vi "Lab Panel V4.90.vi"() -> ()   [LabVIEW 2013] (continued)
                                n569 = local read "TDMS LAB01-2"() -> (w903:refnum<k34>)
                                n570 = Build Array("Testers Name", "Description", "Set Test Cycles", "T-Rise minutes", "T-Rise Deg C") -> (w893:string[])
                                n571 = Unbundle(w892) -> ("NAME"=w891:string, "DESCRIPTION"=w890:string, "CYCLES"=w889:dbl, "T-RISE mins"=w888:dbl, "T-RISE deg C"=w887:dbl)
                                n572 = Number To Decimal String(number=w889) -> (decimal integer string=w902:string)  [unwired: 1 in]
                                n573 = Number To Decimal String(number=w888) -> (decimal integer string=w901:string)  [unwired: 1 in]
                                n574 = Number To Decimal String(number=w887) -> (decimal integer string=w900:string)  [unwired: 1 in]
                                n575 = Build Array(w891, w890, w902, w901, w900) -> (w899:string[])
                                n576 = TDMS Set Properties(5:w899, 7:w893, 11:w903) -> ()  [unwired: 3 in, 4 out]
                              }
                              frame #3 {
                                n577 = local read "DISP LAB01-2"() -> (w905:T4)
                                n578 = Concatenate Strings("LAB01-2  ", w908) -> (w909:string)
                                n579 = Two Button Dialog(message=w909, 1:w906, 2:w907) -> (T button?=w911:bool)
                                n580 = case shown="True" w911 {
                                tunnel: w905 -> [w918 w919]
                                tunnel: [w918 w919] -> w915
                                tunnel: [w917 w920] -> w914
                                tunnel: [w916 w920] -> w913
                                frame False {
                                n581 = Unbundle(w918) -> ("CYCLE"=w917:dbl, "MINS"=w916:dbl)  [unwired: 1 out]
                                }
                                frame True {
                                w920 = 0.0
                                }
                                }
                                n582 = Bundle(cluster=w915, "CYCLE"=w914, "MINS"=w913, "STATUS"="RUN") -> (w904:T4)
                                n583 = local write "DISP LAB01-2"(w904) -> ()
                              }
                              frame #4 {
                                n584 = local read "TEMP START LAB01-2"() -> (w923:cluster{"TL":dbl, "TN":dbl})
                                n585 = Bundle(cluster=w923, "TL"=w921, "TN"=w921) -> (w922:cluster{"TL":dbl, "TN":dbl})
                                n586 = local write "TEMP START LAB01-2"(w922) -> ()
                              }
                            }
                          }
                        }
                      }
                    }
                  }
                }
              }
              event "RUN LAB02-1": Value Change {
                n587 = event-data() -> ("NewVal"=w929:bool)  [unwired: 1 in, 5 out]
                n588 = local read "SIG LAB02-1"() -> (w925:T2)
                n589 = case shown="True" w929 {
                  tunnel: w935 -> [_ w973]
                  tunnel: w934 -> [_ w972]
                  tunnel: w932 -> [w937 w971]
                  tunnel: w933 -> [_ w970]
                  tunnel: w931 -> [_ w969]
                  tunnel: [w936 w968] -> w930
                  tunnel: w928 -> [_ w967]
                  tunnel: w927 -> [_ w966]
                  tunnel: w926 -> [_ w965]
                  tunnel: w925 -> [_ w964]
                  tunnel: w924 -> [_ w963]
                  frame False {
                    # "stop test"
                    n590 = stacked-sequence {
                      tunnel: w937 -> [w946 _]
                      tunnel: [w938 _] -> w936
                      frame #0 {
                        n591 = local read "DISP LAB02-1"() -> (w945:T4)
                        n592 = Unbundle(w945) -> ("CYCLE"=w943:dbl, "MINS"=w944:dbl)  [unwired: 1 out]
                        n593 = case shown="\"CYCLE TEST\"" w946 {
                          tunnel: w944 -> [_ _ w953]
                          tunnel: w943 -> [w951 w952 _]
                          tunnel: [w951 w952 w953] -> w942
                          frame "CHART TEST", Default {
                          }
                          frame "CYCLE TEST" {
                          }
                          frame "T-RISE TEST" {
                          }
                        }
                        n594 = local read "TDMS LAB02-1"() -> (w950:refnum<k34>)
                        n595 = Build Array("STOPPED") -> (w947:string[])
                        n596 = Build Array(w942) -> (w941:dbl[])
                        n597 = TDMS Write(0:w950, 5:"TEST RESULT", 7:w947, 9:w941) -> (4:w939:refnum<k34>, 15:w940:errorcluster)  [unwired: 2 in, 2 out]
                        n598 = TDMS Close(8:w940, 11:w939) -> (0:w938:errorcluster)  [unwired: 1 out]
                      }
                      frame #1 {
                        n599 = local read "DISP LAB02-1"() -> (w957:T4)
                        n600 = stacked-sequence {
                          tunnel: "LAB02-1" -> [w959 w961]
                          frame #0 {
                            n601 = call "sub vi - defrag tdms v1.vi"("panel id"=w959) -> ("error out"=w958:errorcluster)  [unwired: 10 in]
                            n602 = local write "data file error"(w958) -> ()
                          }
                          frame #1 {
                            n603 = local write "RESULT LAB02-1"(FALSE) -> ()
                            n604 = call "Save data file (stop) v3.vi"("panel id"=w961) -> ("network file save error"=w960:errorcluster)  [unwired: 9 in, 1 out]
                            n605 = local write "data file error"(w960) -> ()
                          }
                        }
                        n606 = Bundle(cluster=w957, "STATUS"="STOP") -> (w955:T4)  [unwired: 2 in]
                        n607 = local write "DISP LAB02-1"(w955) -> ()
                      }
                    }
                  }
                  frame True {
                    n608 = stacked-sequence {
                      seq-local: [w975 _] -> [_ w979]
                      tunnel: w973 -> [_ w989]
                      tunnel: w972 -> [_ w988]
                      tunnel: w971 -> [_ w987]
                      tunnel: w970 -> [_ w986]
                      tunnel: w969 -> [_ w985]
                      tunnel: [_ w984] -> w968
                      tunnel: w967 -> [_ w983]
                      tunnel: w966 -> [_ w982]
                      tunnel: w965 -> [_ w981]
                      tunnel: w964 -> [w974 w980]
                      tunnel: w963 -> [_ w978]
                      frame #0 {
                        n609 = Unbundle(w974) -> ("AMPS"=w977:dbl)  [unwired: 4 out]
                        n610 = call "Check For Amps on v1.vi"("ID"="LAB02-1", "amps"=w977) -> ("amps"=w975:bool)  [unwired: 9 in]
                      }
                      frame #1 {
                        n611 = case shown="True" w979 {
                          tunnel: w989 -> [_ w1002]
                          tunnel: w988 -> [_ w1001]
                          tunnel: w987 -> [_ w1000]
                          tunnel: w986 -> [_ w999]
                          tunnel: w985 -> [_ w998]
                          tunnel: [errorcluster {"status"=FALSE, "code"=0, "source"=""} ("error out") w997] -> w984
                          tunnel: w983 -> [_ w996]
                          tunnel: w982 -> [_ w995]
                          tunnel: w981 -> [_ w994]
                          tunnel: w980 -> [_ w993]
                          tunnel: w978 -> [_ w992]
                          frame False {
                            w991 = FALSE
                            n612 = local write "RUN LAB02-1"(w991) -> ()
                            n613 = local write "run lab02-1"(w991) -> ()
                          }
                          frame True {
                            n614 = stacked-sequence {
                              seq-local: [w1003 _ _ _ _] -> [_ w1027 _ _ _]
                              tunnel: w1002 -> [w1008 _ _ _ _]
                              tunnel: w1001 -> [w1005 _ _ _ _]
                              tunnel: w1000 -> [w1018 _ _ _ _]
                              tunnel: w999 -> [w1011 _ _ _ _]
                              tunnel: w998 -> [w1006 _ _ _ _]
                              tunnel: [_ w1022 _ _ _] -> w997
                              tunnel: w996 -> [_ _ _ w1048 _]
                              tunnel: w995 -> [_ _ _ w1047 _]
                              tunnel: w994 -> [_ _ _ w1046 _]
                              tunnel: w993 -> [_ _ _ _ _]
                              tunnel: w992 -> [_ _ _ _ w1062]
                              frame #0 {
                                w1004 = "\\"
                                n615 = local read "SET LAB02-1"() -> (w1013:T5)
                                n616 = case shown="\"CYCLE TEST\"" w1018 {
                                tunnel: ["L02-1-CHART TEST-" "L02-1-CYCLE TEST-" "L02-1-T-RISE TEST-"] -> w1014
                                frame "CHART TEST", Default {
                                }
                                frame "CYCLE TEST" {
                                }
                                frame "T-RISE TEST" {
                                }
                                }
                                n617 = Unbundle(w1013) -> ("DESCRIPTION"=w1012:string)  [unwired: 4 out]
                                n618 = Concatenate Strings(w1008, "\\", w1006, w1004, w1005, w1004) -> (w1015:string)
                                n619 = String To Path(string=w1015) -> (path=w1017:path)
                                n620 = Concatenate Strings(w1015, w1014, w1012, "-", w1011, ".tdms") -> (w1003:string)
                                n621 = Create Folder(path (use dialog)=w1017) -> (error out=w1016:errorcluster)  [unwired: 2 in, 2 out]
                                n622 = global write "Global 1.vi" "LAB02-1 FILE"(w1003) -> ()
                                n623 = call <vilib>:"Clear Errors.vi"("error in (no error)"=w1016) -> ()  [unwired: 6 in, 1 out]
                              }
                              frame #1 {
                                (unwired) FALSE
                                n624 = String To Path(string=w1027) -> (path=w1023:path)
                                n625 = TDMS Open(6:FALSE, 10:T20."create or replace" ("operation (0:open)"), 11:w1023) -> (0:w1022:errorcluster, 3:→"TDMS LAB02-1":refnum<k34>)  [unwired: 4 in]
                              }
                              frame #2 {
                                n626 = local read "SET LAB02-1"() -> (w1033:T5)
                                n627 = local read "TDMS LAB02-1"() -> (w1044:refnum<k34>)
                                n628 = Build Array("Testers Name", "Description", "Set Test Cycles", "T-Rise minutes", "T-Rise Deg C") -> (w1034:string[])
                                n629 = Unbundle(w1033) -> ("NAME"=w1032:string, "DESCRIPTION"=w1031:string, "CYCLES"=w1030:dbl, "T-RISE mins"=w1029:dbl, "T-RISE deg C"=w1028:dbl)
                                n630 = Number To Decimal String(number=w1030) -> (decimal integer string=w1043:string)  [unwired: 1 in]
                                n631 = Number To Decimal String(number=w1029) -> (decimal integer string=w1042:string)  [unwired: 1 in]
                                n632 = Number To Decimal String(number=w1028) -> (decimal integer string=w1041:string)  [unwired: 1 in]
                                n633 = Build Array(w1032, w1031, w1043, w1042, w1041) -> (w1040:string[])
                                n634 = TDMS Set Properties(5:w1040, 7:w1034, 11:w1044) -> ()  [unwired: 3 in, 4 out]
                              }
                              frame #3 {
                                n635 = local read "DISP LAB02-1"() -> (w1049:T4)
                                n636 = Concatenate Strings("LAB02-1  ", w1048) -> (w1050:string)
                                n637 = Two Button Dialog(message=w1050, 1:w1046, 2:w1047) -> (T button?=w1052:bool)
                                n638 = case shown="True" w1052 {
                                tunnel: w1049 -> [w1059 w1060]
                                tunnel: [w1059 w1060] -> w1056
                                tunnel: [w1058 w1061] -> w1055
                                tunnel: [w1057 w1061] -> w1054
                                frame False {
                                n639 = Unbundle(w1059) -> ("CYCLE"=w1058:dbl, "MINS"=w1057:dbl)  [unwired: 1 out]
                                }
                                frame True {
                                w1061 = 0.0
                                }
                                }
                                n640 = Bundle(cluster=w1056, "CYCLE"=w1055, "MINS"=w1054, "STATUS"="RUN") -> (w1045:T4)
                                n641 = local write "DISP LAB02-1"(w1045) -> ()
                              }
                              frame #4 {
                                n642 = local read "TEMP START LAB02-1"() -> (w1064:cluster{"TL":dbl, "TN":dbl})
                                n643 = Bundle(cluster=w1064, "TL"=w1062, "TN"=w1062) -> (w1063:cluster{"TL":dbl, "TN":dbl})
                                n644 = local write "TEMP START LAB02-1"(w1063) -> ()
                              }
                            }
                          }
                        }
                      }
                    }
                  }
                }
                n645 = local write "run lab02-1"(w929) -> ()
              }
              event "RUN LAB02-2": Value Change {
                n646 = event-data() -> ("NewVal"=w1069:bool)  [unwired: 1 in, 5 out]
                n647 = local write "run lab02-2"(w1069) -> ()
                n648 = case shown="True" w1069 {
                  tunnel: w1075 -> [_ w1113]
                  tunnel: w1074 -> [_ w1112]
                  tunnel: w1072 -> [w1077 w1111]
                  tunnel: w1073 -> [_ w1110]
                  tunnel: w1071 -> [_ w1109]
                  tunnel: [w1076 w1108] -> w1070
                  tunnel: w1068 -> [_ w1107]
                  tunnel: w1067 -> [_ w1106]
                  tunnel: w1066 -> [_ w1105]
                  tunnel: w1065 -> [_ w1103]
                  frame False {
                    # "stop test"
                    n649 = stacked-sequence {
                      tunnel: w1077 -> [w1086 _]
                      tunnel: [w1078 _] -> w1076
                      frame #0 {
                        n650 = local read "DISP LAB02-2"() -> (w1085:T4)
                        n651 = Unbundle(w1085) -> ("CYCLE"=w1083:dbl, "MINS"=w1084:dbl)  [unwired: 1 out]
                        n652 = case shown="\"CYCLE TEST\"" w1086 {
                          tunnel: w1084 -> [_ _ w1093]
                          tunnel: w1083 -> [w1091 w1092 _]
                          tunnel: [w1091 w1092 w1093] -> w1082
                          frame "CHART TEST", Default {
                          }
                          frame "CYCLE TEST" {
                          }
                          frame "T-RISE TEST" {
                          }
                        }
                        n653 = local read "TDMS LAB02-2"() -> (w1090:refnum<k34>)
                        n654 = Build Array("STOPPED") -> (w1087:string[])
                        n655 = Build Array(w1082) -> (w1081:dbl[])
                        n656 = TDMS Write(0:w1090, 5:"TEST RESULT", 7:w1087, 9:w1081) -> (4:w1079:refnum<k34>, 15:w1080:errorcluster)  [unwired: 2 in, 2 out]
                        n657 = TDMS Close(8:w1080, 11:w1079) -> (0:w1078:errorcluster)  [unwired: 1 out]
                      }
                      frame #1 {
                        n658 = local read "DISP LAB02-2"() -> (w1097:T4)
                        n659 = stacked-sequence {
                          tunnel: "LAB02-2" -> [w1099 w1101]
                          frame #0 {
                            n660 = call "sub vi - defrag tdms v1.vi"("panel id"=w1099) -> ("error out"=w1098:errorcluster)  [unwired: 10 in]
                            n661 = local write "data file error"(w1098) -> ()
                          }
                          frame #1 {
                            n662 = call "Save data file (stop) v3.vi"("panel id"=w1101) -> ("network file save error"=w1100:errorcluster)  [unwired: 9 in, 1 out]
                            n663 = local write "RESULT LAB02-2"(FALSE) -> ()
                            n664 = local write "data file error"(w1100) -> ()
                          }
                        }
                        n665 = Bundle(cluster=w1097, "STATUS"="STOP") -> (w1095:T4)  [unwired: 2 in]
                        n666 = local write "DISP LAB02-2"(w1095) -> ()
                      }
                    }
                  }
                  frame True {
                    n667 = local read "SIG LAB02-2"() -> (w1104:T2)
                    n668 = stacked-sequence {
                      seq-local: [w1115 _] -> [_ w1119]
                      tunnel: w1113 -> [_ w1129]
                      tunnel: w1112 -> [_ w1128]
                      tunnel: w1111 -> [_ w1127]
                      tunnel: w1110 -> [_ w1126]
                      tunnel: w1109 -> [_ w1125]
                      tunnel: [_ w1124] -> w1108
                      tunnel: w1107 -> [_ w1123]
                      tunnel: w1106 -> [_ w1122]
                      tunnel: w1105 -> [_ w1121]
                      tunnel: w1104 -> [w1114 w1120]
                      tunnel: w1103 -> [_ w1118]
                      frame #0 {
                        n669 = Unbundle(w1114) -> ("AMPS"=w1117:dbl)  [unwired: 4 out]
                        n670 = call "Check For Amps on v1.vi"("ID"="LAB02-2", "amps"=w1117) -> ("amps"=w1115:bool)  [unwired: 9 in]
                      }
                      frame #1 {
                        n671 = case shown="True" w1119 {
                          tunnel: w1129 -> [_ w1142]
                          tunnel: w1128 -> [_ w1141]
                          tunnel: w1127 -> [_ w1140]
                          tunnel: w1126 -> [_ w1139]
                          tunnel: w1125 -> [_ w1138]
                          tunnel: [errorcluster {"status"=FALSE, "code"=0, "source"=""} ("error out") w1137] -> w1124
                          tunnel: w1123 -> [_ w1136]
                          tunnel: w1122 -> [_ w1135]
                          tunnel: w1121 -> [_ w1134]
                          tunnel: w1120 -> [_ w1133]
                          tunnel: w1118 -> [_ w1132]
                          frame False {
                            w1130 = FALSE
                            n672 = local write "RUN LAB02-2"(w1130) -> ()
                            n673 = local write "run lab02-2"(w1130) -> ()
                          }
                          frame True {
                            n674 = stacked-sequence {
                              seq-local: [w1143 _ _ _ _] -> [_ w1167 _ _ _]
                              tunnel: w1142 -> [w1148 _ _ _ _]
                              tunnel: w1141 -> [w1145 _ _ _ _]
                              tunnel: w1140 -> [w1158 _ _ _ _]
                              tunnel: w1139 -> [w1151 _ _ _ _]
                              tunnel: w1138 -> [w1146 _ _ _ _]
                              tunnel: [_ w1162 _ _ _] -> w1137
                              tunnel: w1136 -> [_ _ _ w1188 _]
                              tunnel: w1135 -> [_ _ _ w1187 _]
                              tunnel: w1134 -> [_ _ _ w1186 _]
                              tunnel: w1133 -> [_ _ _ _ _]
                              tunnel: w1132 -> [_ _ _ _ w1202]
                              frame #0 {
                                w1144 = "\\"
                                n675 = local read "SET LAB02-2"() -> (w1153:T5)
                                n676 = case shown="\"CYCLE TEST\"" w1158 {
                                tunnel: ["L02-2-CHART TEST-" "L02-2-CYCLE TEST-" "L02-2-T-RISE TEST-"] -> w1154
                                frame "CHART TEST", Default {
                                }
                                frame "CYCLE TEST" {
                                }
                                frame "T-RISE TEST" {
                                }
                                }
                                n677 = Unbundle(w1153) -> ("DESCRIPTION"=w1152:string)  [unwired: 4 out]
                                n678 = Concatenate Strings(w1148, "\\", w1146, w1144, w1145, w1144) -> (w1155:string)
                                n679 = String To Path(string=w1155) -> (path=w1157:path)
                                n680 = Concatenate Strings(w1155, w1154, w1152, "-", w1151, ".tdms") -> (w1143:string)
                                n681 = Create Folder(path (use dialog)=w1157) -> (error out=w1156:errorcluster)  [unwired: 2 in, 2 out]
                                n682 = global write "Global 1.vi" "LAB02-2 FILE"(w1143) -> ()
                                n683 = call <vilib>:"Clear Errors.vi"("error in (no error)"=w1156) -> ()  [unwired: 6 in, 1 out]
                              }
                              frame #1 {
                                (unwired) FALSE
                                n684 = String To Path(string=w1167) -> (path=w1163:path)
                                n685 = TDMS Open(6:FALSE, 10:T20."create or replace" ("operation (0:open)"), 11:w1163) -> (0:w1162:errorcluster, 3:→"TDMS LAB02-2":refnum<k34>)  [unwired: 4 in]
                              }
                              frame #2 {
                                n686 = local read "SET LAB02-2"() -> (w1173:T5)
                                n687 = local read "TDMS LAB02-2"() -> (w1184:refnum<k34>)
                                n688 = Build Array("Testers Name", "Description", "Set Test Cycles", "T-Rise minutes", "T-Rise Deg C") -> (w1174:string[])
                                n689 = Unbundle(w1173) -> ("NAME"=w1172:string, "DESCRIPTION"=w1171:string, "CYCLES"=w1170:dbl, "T-RISE mins"=w1169:dbl, "T-RISE deg C"=w1168:dbl)
                                n690 = Number To Decimal String(number=w1170) -> (decimal integer string=w1183:string)  [unwired: 1 in]
                                n691 = Number To Decimal String(number=w1169) -> (decimal integer string=w1182:string)  [unwired: 1 in]
                                n692 = Number To Decimal String(number=w1168) -> (decimal integer string=w1181:string)  [unwired: 1 in]
                                n693 = Build Array(w1172, w1171, w1183, w1182, w1181) -> (w1180:string[])
                                n694 = TDMS Set Properties(5:w1180, 7:w1174, 11:w1184) -> ()  [unwired: 3 in, 4 out]
                              }
                              frame #3 {
                                n695 = local read "DISP LAB02-2"() -> (w1189:T4)
                                n696 = Concatenate Strings("LAB02-2  ", w1188) -> (w1190:string)
                                n697 = Two Button Dialog(message=w1190, 1:w1186, 2:w1187) -> (T button?=w1192:bool)
                                n698 = case shown="True" w1192 {
                                tunnel: w1189 -> [w1199 w1200]
                                tunnel: [w1199 w1200] -> w1196
                                tunnel: [w1198 w1201] -> w1195
                                tunnel: [w1197 w1201] -> w1194
                                frame False {
                                n699 = Unbundle(w1199) -> ("CYCLE"=w1198:dbl, "MINS"=w1197:dbl)  [unwired: 1 out]
                                }
                                frame True {
                                w1201 = 0.0
                                }
                                }
                                n700 = Bundle(cluster=w1196, "CYCLE"=w1195, "MINS"=w1194, "STATUS"="RUN") -> (w1185:T4)
                                n701 = local write "DISP LAB02-2"(w1185) -> ()
                              }
                              frame #4 {
                                n702 = local read "TEMP START LAB02-2"() -> (w1204:cluster{"TL":dbl, "TN":dbl})
                                n703 = Bundle(cluster=w1204, "TL"=w1202, "TN"=w1202) -> (w1203:cluster{"TL":dbl, "TN":dbl})
                                n704 = local write "TEMP START LAB02-2"(w1203) -> ()
                              }
                            }
                          }
                        }
                      }
                    }
                  }
                }
              }
              event "RUN LAB03-1": Value Change {
                n705 = event-data() -> ("NewVal"=w1209:bool)  [unwired: 1 in, 5 out]
                n706 = local write "run lab03-1"(w1209) -> ()
                n707 = case shown="True" w1209 {
                  tunnel: w1215 -> [_ w1253]
                  tunnel: w1214 -> [_ w1252]
                  tunnel: w1212 -> [w1217 w1251]
                  tunnel: w1213 -> [_ w1250]
                  tunnel: w1211 -> [_ w1249]
                  tunnel: [w1216 w1248] -> w1210
                  tunnel: w1208 -> [_ w1247]
                  tunnel: w1207 -> [_ w1246]
                  tunnel: w1206 -> [_ w1245]
                  tunnel: w1205 -> [_ w1243]
                  frame False {
                    # "stop test"
                    n708 = stacked-sequence {
                      tunnel: w1217 -> [w1226 _]
                      tunnel: [w1218 _] -> w1216
                      frame #0 {
                        n709 = local read "DISP LAB03-1"() -> (w1225:T4)
                        n710 = Unbundle(w1225) -> ("CYCLE"=w1223:dbl, "MINS"=w1224:dbl)  [unwired: 1 out]
                        n711 = case shown="\"CYCLE TEST\"" w1226 {
                          tunnel: w1224 -> [_ _ w1233]
                          tunnel: w1223 -> [w1231 w1232 _]
                          tunnel: [w1231 w1232 w1233] -> w1222
                          frame "CHART TEST", Default {
                          }
                          frame "CYCLE TEST" {
                          }
                          frame "T-RISE TEST" {
                          }
                        }
                        n712 = local read "TDMS LAB03-1"() -> (w1230:refnum<k34>)
                        n713 = Build Array("STOPPED") -> (w1227:string[])
                        n714 = Build Array(w1222) -> (w1221:dbl[])
                        n715 = TDMS Write(0:w1230, 5:"TEST RESULT", 7:w1227, 9:w1221) -> (4:w1219:refnum<k34>, 15:w1220:errorcluster)  [unwired: 2 in, 2 out]
                        n716 = TDMS Close(8:w1220, 11:w1219) -> (0:w1218:errorcluster)  [unwired: 1 out]
                      }
                      frame #1 {
                        n717 = local read "DISP LAB03-1"() -> (w1237:T4)
                        n718 = stacked-sequence {
                          tunnel: "LAB03-1" -> [w1239 w1241]
                          frame #0 {
                            n719 = call "sub vi - defrag tdms v1.vi"("panel id"=w1239) -> ("error out"=w1238:errorcluster)  [unwired: 10 in]
                            n720 = local write "data file error"(w1238) -> ()
                          }
                          frame #1 {
                            n721 = call "Save data file (stop) v3.vi"("panel id"=w1241) -> ("network file save error"=w1240:errorcluster)  [unwired: 9 in, 1 out]
                            n722 = local write "RESULT LAB03-1"(FALSE) -> ()
                            n723 = local write "data file error"(w1240) -> ()
                          }
                        }
                        n724 = Bundle(cluster=w1237, "STATUS"="STOP") -> (w1235:T4)  [unwired: 2 in]
                        n725 = local write "DISP LAB03-1"(w1235) -> ()
                      }
                    }
                  }
                  frame True {
                    n726 = local read "SIG LAB03-1"() -> (w1244:T2)
                    n727 = stacked-sequence {
                      seq-local: [w1255 _] -> [_ w1259]
                      tunnel: w1253 -> [_ w1269]
                      tunnel: w1252 -> [_ w1268]
                      tunnel: w1251 -> [_ w1267]
                      tunnel: w1250 -> [_ w1266]
                      tunnel: w1249 -> [_ w1265]
                      tunnel: [_ w1264] -> w1248
                      tunnel: w1247 -> [_ w1263]
                      tunnel: w1246 -> [_ w1262]
                      tunnel: w1245 -> [_ w1261]
                      tunnel: w1244 -> [w1254 w1260]
                      tunnel: w1243 -> [_ w1258]
                      frame #0 {
                        n728 = Unbundle(w1254) -> ("AMPS"=w1257:dbl)  [unwired: 4 out]
                        n729 = call "Check For Amps on v1.vi"("ID"="LAB03-1", "amps"=w1257) -> ("amps"=w1255:bool)  [unwired: 9 in]
                      }
                      frame #1 {
                        n730 = case shown="True" w1259 {
                          tunnel: w1269 -> [_ w1282]
                          tunnel: w1268 -> [_ w1281]
                          tunnel: w1267 -> [_ w1280]
                          tunnel: w1266 -> [_ w1279]
                          tunnel: w1265 -> [_ w1278]
                          tunnel: [errorcluster {"status"=FALSE, "code"=0, "source"=""} ("error out") w1277] -> w1264
                          tunnel: w1263 -> [_ w1276]
                          tunnel: w1262 -> [_ w1275]
                          tunnel: w1261 -> [_ w1274]
                          tunnel: w1260 -> [_ w1273]
                          tunnel: w1258 -> [_ w1272]
                          frame False {
                            w1270 = FALSE
                            n731 = local write "RUN LAB03-1"(w1270) -> ()
                            n732 = local write "run lab03-1"(w1270) -> ()
                          }
                          frame True {
                            n733 = stacked-sequence {
                              seq-local: [w1283 _ _ _ _] -> [_ w1307 _ _ _]
                              tunnel: w1282 -> [w1288 _ _ _ _]
                              tunnel: w1281 -> [w1285 _ _ _ _]
                              tunnel: w1280 -> [w1298 _ _ _ _]
                              tunnel: w1279 -> [w1291 _ _ _ _]
                              tunnel: w1278 -> [w1286 _ _ _ _]
                              tunnel: [_ w1302 _ _ _] -> w1277
                              tunnel: w1276 -> [_ _ _ w1327 _]
                              tunnel: w1275 -> [_ _ _ w1326 _]
                              tunnel: w1274 -> [_ _ _ w1325 _]
                              tunnel: w1273 -> [_ _ _ _ _]
                              tunnel: w1272 -> [_ _ _ _ w1342]
                              frame #0 {
                                w1284 = "\\"
                                n734 = local read "SET LAB03-1"() -> (w1293:T5)
                                n735 = case shown="\"T-RISE TEST\"" w1298 {
                                tunnel: ["L03-1-CHART TEST-" "L03-1-CYCLE TEST-" "L03-1-T-RISE TEST-"] -> w1294
                                frame "CHART TEST", Default {
                                }
                                frame "CYCLE TEST" {
                                }
                                frame "T-RISE TEST" {
                                }
                                }
                                n736 = Unbundle(w1293) -> ("DESCRIPTION"=w1292:string)  [unwired: 4 out]
                                n737 = Concatenate Strings(w1288, "\\", w1286, w1284, w1285, w1284) -> (w1295:string)
                                n738 = String To Path(string=w1295) -> (path=w1297:path)
                                n739 = Concatenate Strings(w1295, w1294, w1292, "-", w1291, ".tdms") -> (w1283:string)
                                n740 = Create Folder(path (use dialog)=w1297) -> (error out=w1296:errorcluster)  [unwired: 2 in, 2 out]
                                n741 = global write "Global 1.vi" "LAB03-1 FILE"(w1283) -> ()
                                n742 = call <vilib>:"Clear Errors.vi"("error in (no error)"=w1296) -> ()  [unwired: 6 in, 1 out]
                              }
                              frame #1 {
                                (unwired) FALSE
                                n743 = String To Path(string=w1307) -> (path=w1303:path)
                                n744 = TDMS Open(6:FALSE, 10:T20."create or replace" ("operation (0:open)"), 11:w1303) -> (0:w1302:errorcluster, 3:→"TDMS LAB03-1":refnum<k34>)  [unwired: 4 in]
                              }
                              frame #2 {
                                n745 = local read "SET LAB03-1"() -> (w1313:T5)
                                n746 = local read "TDMS LAB03-1"() -> (w1324:refnum<k34>)
                                n747 = Build Array("Testers Name", "Description", "Set Test Cycles", "T-Rise minutes", "T-Rise Deg C") -> (w1314:string[])
                                n748 = Unbundle(w1313) -> ("NAME"=w1312:string, "DESCRIPTION"=w1311:string, "CYCLES"=w1310:dbl, "T-RISE mins"=w1309:dbl, "T-RISE deg C"=w1308:dbl)
                                n749 = Number To Decimal String(number=w1310) -> (decimal integer string=w1323:string)  [unwired: 1 in]
                                n750 = Number To Decimal String(number=w1309) -> (decimal integer string=w1322:string)  [unwired: 1 in]
                                n751 = Number To Decimal String(number=w1308) -> (decimal integer string=w1321:string)  [unwired: 1 in]
                                n752 = Build Array(w1312, w1311, w1323, w1322, w1321) -> (w1320:string[])
                                n753 = TDMS Set Properties(5:w1320, 7:w1314, 11:w1324) -> ()  [unwired: 3 in, 4 out]
                              }
                              frame #3 {
                                n754 = local read "DISP LAB03-1"() -> (w1329:T4)
                                n755 = Concatenate Strings("LAB03-1  ", w1327) -> (w1330:string)
                                n756 = Two Button Dialog(message=w1330, 1:w1325, 2:w1326) -> (T button?=w1332:bool)
                                n757 = case shown="True" w1332 {
                                tunnel: w1329 -> [w1339 w1340]
                                tunnel: [w1339 w1340] -> w1336
                                tunnel: [w1338 w1341] -> w1335
                                tunnel: [w1337 w1341] -> w1334
                                frame False {
                                n758 = Unbundle(w1339) -> ("CYCLE"=w1338:dbl, "MINS"=w1337:dbl)  [unwired: 1 out]
                                }
                                frame True {
                                w1341 = 0.0
                                }
                                }
                                n759 = Bundle(cluster=w1336, "CYCLE"=w1335, "MINS"=w1334, "STATUS"="RUN") -> (w1328:T4)
                                n760 = local write "DISP LAB03-1"(w1328) -> ()
                              }
                              frame #4 {
                                n761 = local read "TEMP START LAB03-1"() -> (w1344:cluster{"TL":dbl, "TN":dbl})
                                n762 = Bundle(cluster=w1344, "TL"=w1342, "TN"=w1342) -> (w1343:cluster{"TL":dbl, "TN":dbl})
                                n763 = local write "TEMP START LAB03-1"(w1343) -> ()
                              }
                            }
                          }
                        }
                      }
                    }
                  }
                }
              }
              event "RUN LAB03-2": Value Change {
                n764 = event-data() -> ("NewVal"=w1349:bool)  [unwired: 1 in, 5 out]
                n765 = local write "run lab03-2"(w1349) -> ()
                n766 = case shown="True" w1349 {
                  tunnel: w1355 -> [_ w1393]
                  tunnel: w1354 -> [_ w1392]
                  tunnel: w1352 -> [w1357 w1391]
                  tunnel: w1353 -> [_ w1390]
                  tunnel: w1351 -> [_ w1389]
                  tunnel: [w1356 w1388] -> w1350
                  tunnel: w1348 -> [_ w1387]
                  tunnel: w1347 -> [_ w1386]
                  tunnel: w1346 -> [_ w1385]
                  tunnel: w1345 -> [_ w1383]
                  frame False {
                    # "stop test"
                    n767 = stacked-sequence {
                      tunnel: w1357 -> [w1366 _]
                      tunnel: [w1358 _] -> w1356
                      frame #0 {
                        n768 = local read "DISP LAB03-2"() -> (w1365:T4)
                        n769 = Unbundle(w1365) -> ("CYCLE"=w1363:dbl, "MINS"=w1364:dbl)  [unwired: 1 out]
                        n770 = case shown="\"CYCLE TEST\"" w1366 {
                          tunnel: w1364 -> [_ _ w1373]
                          tunnel: w1363 -> [w1371 w1372 _]
                          tunnel: [w1371 w1372 w1373] -> w1362
                          frame "CHART TEST", Default {
                          }
                          frame "CYCLE TEST" {
                          }
                          frame "T-RISE TEST" {
                          }
                        }
                        n771 = local read "TDMS LAB03-2"() -> (w1370:refnum<k34>)
                        n772 = Build Array("STOPPED") -> (w1367:string[])
                        n773 = Build Array(w1362) -> (w1361:dbl[])
                        n774 = TDMS Write(0:w1370, 5:"TEST RESULT", 7:w1367, 9:w1361) -> (4:w1359:refnum<k34>, 15:w1360:errorcluster)  [unwired: 2 in, 2 out]
                        n775 = TDMS Close(8:w1360, 11:w1359) -> (0:w1358:errorcluster)  [unwired: 1 out]
                      }
                      frame #1 {
                        n776 = local read "DISP LAB03-2"() -> (w1377:T4)
                        n777 = stacked-sequence {
                          tunnel: "LAB03-2" -> [w1379 w1381]
                          frame #0 {
                            n778 = call "sub vi - defrag tdms v1.vi"("panel id"=w1379) -> ("error out"=w1378:errorcluster)  [unwired: 10 in]
                            n779 = local write "data file error"(w1378) -> ()
                          }
                          frame #1 {
                            n780 = call "Save data file (stop) v3.vi"("panel id"=w1381) -> ("network file save error"=w1380:errorcluster)  [unwired: 9 in, 1 out]
                            n781 = local write "RESULT LAB03-2"(FALSE) -> ()
                            n782 = local write "data file error"(w1380) -> ()
                          }
                        }
                        n783 = Bundle(cluster=w1377, "STATUS"="STOP") -> (w1375:T4)  [unwired: 2 in]
                        n784 = local write "DISP LAB03-2"(w1375) -> ()
                      }
                    }
                  }
                  frame True {
                    n785 = local read "SIG LAB03-2"() -> (w1384:T2)
                    n786 = stacked-sequence {
                      seq-local: [w1395 _] -> [_ w1399]
                      tunnel: w1393 -> [_ w1409]
                      tunnel: w1392 -> [_ w1408]
                      tunnel: w1391 -> [_ w1407]
                      tunnel: w1390 -> [_ w1406]
                      tunnel: w1389 -> [_ w1405]
                      tunnel: [_ w1404] -> w1388
                      tunnel: w1387 -> [_ w1403]
                      tunnel: w1386 -> [_ w1402]
                      tunnel: w1385 -> [_ w1401]
                      tunnel: w1384 -> [w1394 w1400]
                      tunnel: w1383 -> [_ w1398]
                      frame #0 {
                        n787 = Unbundle(w1394) -> ("AMPS"=w1397:dbl)  [unwired: 4 out]
                        n788 = call "Check For Amps on v1.vi"("ID"="LAB03-2", "amps"=w1397) -> ("amps"=w1395:bool)  [unwired: 9 in]
                      }
                      frame #1 {
                        n789 = case shown="True" w1399 {
                          tunnel: w1409 -> [_ w1422]
                          tunnel: w1408 -> [_ w1421]
                          tunnel: w1407 -> [_ w1420]
                          tunnel: w1406 -> [_ w1419]
                          tunnel: w1405 -> [_ w1418]
                          tunnel: [errorcluster {"status"=FALSE, "code"=0, "source"=""} ("error out") w1417] -> w1404
                          tunnel: w1403 -> [_ w1416]
                          tunnel: w1402 -> [_ w1415]
                          tunnel: w1401 -> [_ w1414]
                          tunnel: w1400 -> [_ w1413]
                          tunnel: w1398 -> [_ w1412]
                          frame False {
                            w1410 = FALSE
                            n790 = local write "RUN LAB03-2"(w1410) -> ()
                            n791 = local write "run lab03-2"(w1410) -> ()
                          }
                          frame True {
                            n792 = stacked-sequence {
                              seq-local: [w1423 _ _ _ _] -> [_ w1447 _ _ _]
                              tunnel: w1422 -> [w1428 _ _ _ _]
                              tunnel: w1421 -> [w1425 _ _ _ _]
                              tunnel: w1420 -> [w1438 _ _ _ _]
                              tunnel: w1419 -> [w1431 _ _ _ _]
                              tunnel: w1418 -> [w1426 _ _ _ _]
                              tunnel: [_ w1442 _ _ _] -> w1417
                              tunnel: w1416 -> [_ _ _ w1468 _]
                              tunnel: w1415 -> [_ _ _ w1467 _]
                              tunnel: w1414 -> [_ _ _ w1466 _]
                              tunnel: w1413 -> [_ _ _ _ _]
                              tunnel: w1412 -> [_ _ _ _ w1482]
                              frame #0 {
                                w1424 = "\\"
                                n793 = local read "SET LAB03-2"() -> (w1433:T5)
                                n794 = case shown="\"T-RISE TEST\"" w1438 {
                                tunnel: ["L03-2-CHART TEST-" "L03-2-CYCLE TEST-" "L03-2-T-RISE TEST-"] -> w1434
                                frame "CHART TEST", Default {
                                }
                                frame "CYCLE TEST" {
                                }
                                frame "T-RISE TEST" {
                                }
                                }
                                n795 = Unbundle(w1433) -> ("DESCRIPTION"=w1432:string)  [unwired: 4 out]
                                n796 = Concatenate Strings(w1428, "\\", w1426, w1424, w1425, w1424) -> (w1435:string)
                                n797 = String To Path(string=w1435) -> (path=w1437:path)
                                n798 = Concatenate Strings(w1435, w1434, w1432, "-", w1431, ".tdms") -> (w1423:string)
                                n799 = Create Folder(path (use dialog)=w1437) -> (error out=w1436:errorcluster)  [unwired: 2 in, 2 out]
                                n800 = global write "Global 1.vi" "LAB03-2 FILE"(w1423) -> ()
                                n801 = call <vilib>:"Clear Errors.vi"("error in (no error)"=w1436) -> ()  [unwired: 6 in, 1 out]
                              }
                              frame #1 {
                                (unwired) FALSE
                                n802 = String To Path(string=w1447) -> (path=w1443:path)
                                n803 = TDMS Open(6:FALSE, 10:T20."create or replace" ("operation (0:open)"), 11:w1443) -> (0:w1442:errorcluster, 3:→"TDMS LAB03-2":refnum<k34>)  [unwired: 4 in]
                              }
                              frame #2 {
                                n804 = local read "SET LAB03-2"() -> (w1453:T5)
                                n805 = local read "TDMS LAB03-2"() -> (w1464:refnum<k34>)
                                n806 = Build Array("Testers Name", "Description", "Set Test Cycles", "T-Rise minutes", "T-Rise Deg C") -> (w1454:string[])
                                n807 = Unbundle(w1453) -> ("NAME"=w1452:string, "DESCRIPTION"=w1451:string, "CYCLES"=w1450:dbl, "T-RISE mins"=w1449:dbl, "T-RISE deg C"=w1448:dbl)
                                n808 = Number To Decimal String(number=w1450) -> (decimal integer string=w1463:string)  [unwired: 1 in]
                                n809 = Number To Decimal String(number=w1449) -> (decimal integer string=w1462:string)  [unwired: 1 in]
                                n810 = Number To Decimal String(number=w1448) -> (decimal integer string=w1461:string)  [unwired: 1 in]
                                n811 = Build Array(w1452, w1451, w1463, w1462, w1461) -> (w1460:string[])
                                n812 = TDMS Set Properties(5:w1460, 7:w1454, 11:w1464) -> ()  [unwired: 3 in, 4 out]
                              }
                              frame #3 {
                                n813 = local read "DISP LAB03-2"() -> (w1469:T4)
                                n814 = Concatenate Strings("LAB03-2  ", w1468) -> (w1470:string)
                                n815 = Two Button Dialog(message=w1470, 1:w1466, 2:w1467) -> (T button?=w1472:bool)
                                n816 = case shown="True" w1472 {
                                tunnel: w1469 -> [w1479 w1480]
                                tunnel: [w1479 w1480] -> w1476
                                tunnel: [w1478 w1481] -> w1475
                                tunnel: [w1477 w1481] -> w1474
                                frame False {
                                n817 = Unbundle(w1479) -> ("CYCLE"=w1478:dbl, "MINS"=w1477:dbl)  [unwired: 1 out]
                                }
                                frame True {
                                w1481 = 0.0
                                }
                                }
                                n818 = Bundle(cluster=w1476, "CYCLE"=w1475, "MINS"=w1474, "STATUS"="RUN") -> (w1465:T4)
                                n819 = local write "DISP LAB03-2"(w1465) -> ()
                              }
                              frame #4 {
                                n820 = local read "TEMP START LAB03-2"() -> (w1484:cluster{"TL":dbl, "TN":dbl})
                                n821 = Bundle(cluster=w1484, "TL"=w1482, "TN"=w1482) -> (w1483:cluster{"TL":dbl, "TN":dbl})
                                n822 = local write "TEMP START LAB03-2"(w1483) -> ()
                              }
                            }
                          }
                        }
                      }
                    }
                  }
                }
              }
              event "RUN LAB04-1": Value Change {
                n823 = event-data() -> ("NewVal"=w1489:bool)  [unwired: 1 in, 5 out]
                n824 = local write "run lab04-1"(w1489) -> ()
                n825 = case shown="True" w1489 {
                  tunnel: w1495 -> [_ w1533]
                  tunnel: w1494 -> [_ w1532]
                  tunnel: w1492 -> [w1497 w1531]
                  tunnel: w1493 -> [_ w1530]
                  tunnel: w1491 -> [_ w1529]
                  tunnel: [w1496 w1528] -> w1490
                  tunnel: w1488 -> [_ w1527]
                  tunnel: w1487 -> [_ w1526]
                  tunnel: w1486 -> [_ w1525]
                  tunnel: w1485 -> [_ w1523]
                  frame False {
                    # "stop test"
                    n826 = stacked-sequence {
                      tunnel: w1497 -> [w1506 _]
                      tunnel: [w1498 _] -> w1496
                      frame #0 {
                        n827 = local read "DISP LAB04-1"() -> (w1505:T4)
                        n828 = Unbundle(w1505) -> ("CYCLE"=w1503:dbl, "MINS"=w1504:dbl)  [unwired: 1 out]
                        n829 = case shown="\"CYCLE TEST\"" w1506 {
                          tunnel: w1504 -> [_ _ w1513]
                          tunnel: w1503 -> [w1511 w1512 _]
                          tunnel: [w1511 w1512 w1513] -> w1502
                          frame "CHART TEST", Default {
                          }
                          frame "CYCLE TEST" {
                          }
                          frame "T-RISE TEST" {
                          }
                        }
                        n830 = local read "TDMS LAB04-1"() -> (w1510:refnum<k34>)
                        n831 = Build Array("STOPPED") -> (w1507:string[])
                        n832 = Build Array(w1502) -> (w1501:dbl[])
                        n833 = TDMS Write(0:w1510, 5:"TEST RESULT", 7:w1507, 9:w1501) -> (4:w1499:refnum<k34>, 15:w1500:errorcluster)  [unwired: 2 in, 2 out]
                        n834 = TDMS Close(8:w1500, 11:w1499) -> (0:w1498:errorcluster)  [unwired: 1 out]
                      }
                      frame #1 {
                        n835 = local read "DISP LAB04-1"() -> (w1517:T4)
                        n836 = stacked-sequence {
                          tunnel: "LAB04-1" -> [w1519 w1521]
                          frame #0 {
                            n837 = call "sub vi - defrag tdms v1.vi"("panel id"=w1519) -> ("error out"=w1518:errorcluster)  [unwired: 10 in]
                            n838 = local write "data file error"(w1518) -> ()
                          }
                          frame #1 {
                            n839 = call "Save data file (stop) v3.vi"("panel id"=w1521) -> ("network file save error"=w1520:errorcluster)  [unwired: 9 in, 1 out]
                            n840 = local write "RESULT LAB04-1"(FALSE) -> ()
                            n841 = local write "data file error"(w1520) -> ()
                          }
                        }
                        n842 = Bundle(cluster=w1517, "STATUS"="STOP") -> (w1515:T4)  [unwired: 2 in]
                        n843 = local write "DISP LAB04-1"(w1515) -> ()
                      }
                    }
                  }
                  frame True {
